vi "Create Sorted Range.vi"(1 "b":u32, 2 "a":u32) -> (0 "Sorted Range":u32[](array[numeric]))   [LabVIEW 2012]
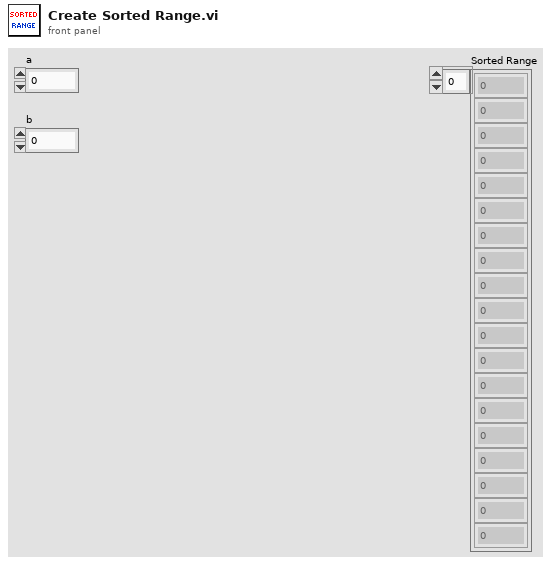
[diagram p1: front panel]
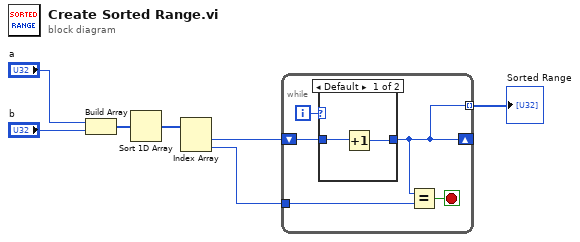
[diagram p0: block diagram]
diagram:
  n1 = Build Array("a", "b") -> (w7:u32[])
  n2 = Sort 1D Array(array=w7) -> (sorted array=w6:u32[])
  n3 = Index Array(array=w6) -> (element #1=w3:u32, element #2=w2:u32)  [unwired: 2 in]
  n4 = while {
    tunnel: w2 -> [w10]
    shift-right: [w8] -> _
    shift-left: w3 -> [w11]
    tunnel: [w8] -> w1 mode=indexing
    i -> [w12]
    stop <- w9 stop-if-true
    n5 = case shown="Default" w12 {
      tunnel: w11 -> [w14 w15]
      tunnel: [w13 w15] -> w8
      frame Default {
        n6 = Increment(x=w14) -> (x+1=w13:u32)
      }
      frame 0 {
      }
    }
    n7 = Equal?(x=w8, y=w10) -> (x = y?=w9:bool)
  }
  "Sorted Range" <- w1
